vi "niRFUtil WFM Multiply Waveforms (real wfm).vi"(2 "Waveform 2 In":T1 {"y" min=0 max=127 format="%.2f"; "dx" format="%^.2e"; "x0" format="%^.2e"}, 3 "Waveform 1 In":T1 {"y" min=0 max=127 format="%.2f"; "dx" format="%^.2e"; "x0" format="%^.2e"}) -> (1 "Waveform Out":T1 {"y" min=0 max=127 format="%.2f"; "dx" format="%^.2e"; "x0" format="%^.2e"})   [LabVIEW 2015, in "niRFUtil.lvlib"]
doc: "(c) Copyright 2006, National Instruments, Inc. This VI may not be duplicated, sold, or distributed without written consent from National Instruments."
uses:
  niRFUtil.lvlib
  Includes/niRFUtil INC Real Waveform.ctl
  Includes/niRFUtil INC Real Array.ctl
  niRFUtil WFM Parse Waveform - Duration (real wfm).vi
  Measurements/niRFUtil MEAS Waveform Statistics (real wfm).vi
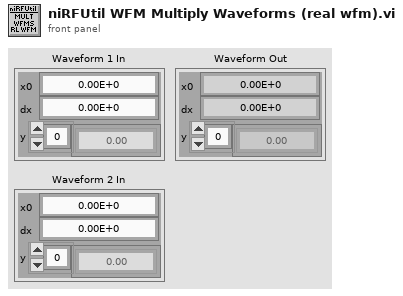
[diagram p1: front panel]
types:
  T1 = typedef "niRFUtil.lvlib/niRFUtil INC Real Waveform.ctl" = cluster{"x0":dbl, "dx":dbl, "y":T2}
  T2 = typedef "niRFUtil.lvlib/niRFUtil INC Real Array.ctl" = sgl[]
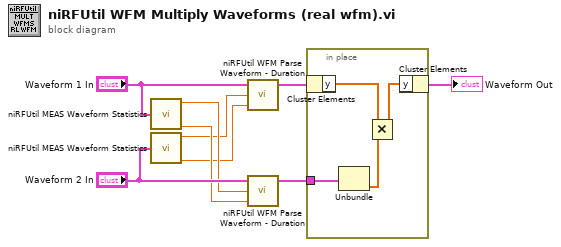
[diagram p0: block diagram]
diagram:
  n1 = call-poly "niRFUtil MEAS Waveform Statistics.vi"("Waveform In"="Waveform 1 In") -> ("Start"=w8:dbl, "Duration"=w7:dbl)  [unwired: 6 out]
  n2 = call-poly "niRFUtil MEAS Waveform Statistics.vi"("Waveform In"="Waveform 2 In") -> ("Start"=w5:dbl, "Duration"=w4:dbl)  [unwired: 6 out]
  n3 = call-poly "niRFUtil WFM Parse Waveform - Duration.vi"("Duration (Inf)"=w4, "Start (-Inf)"=w5, "Waveform In"="Waveform 1 In") -> ("Waveform Out"=w2:T1)  [unwired: 2 out]
  n4 = call-poly "niRFUtil WFM Parse Waveform - Duration.vi"("Duration (Inf)"=w7, "Start (-Inf)"=w8, "Waveform In"="Waveform 2 In") -> ("Waveform Out"=w3:T1)  [unwired: 2 out]
  n5 = in-place {
    in-place-border: w3 -> [w13]
    n6 = in-place-cluster #1(w2) -> ("y"=w11:T2)
    n7 = Unbundle(w13) -> ("y"=w12:T2)  [unwired: 2 out]
    n8 = Multiply(x=w11, y=w12) -> (x*y=w10:T2)
    n9 = in-place-cluster #1("y"=w10) -> (→"Waveform Out":T1)
  }
